vi "cRIO_MAC.vi"() -> (0 "MAC Address":string, 1 "Personality":string)   [LabVIEW 2016]
panel:
  out "File Text":string
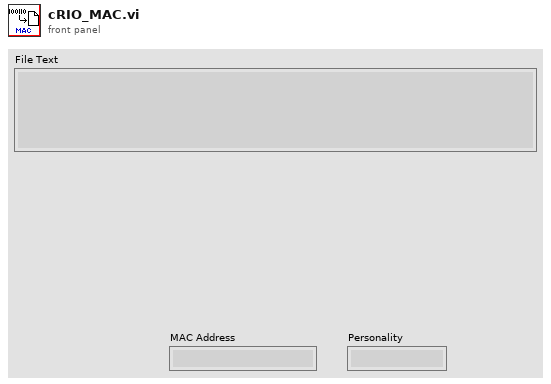
[diagram p1: front panel]
types:
  T1 = enum16{"open", "replace", "create", "open or create", "replace or create", "replace or create with confirmation"}
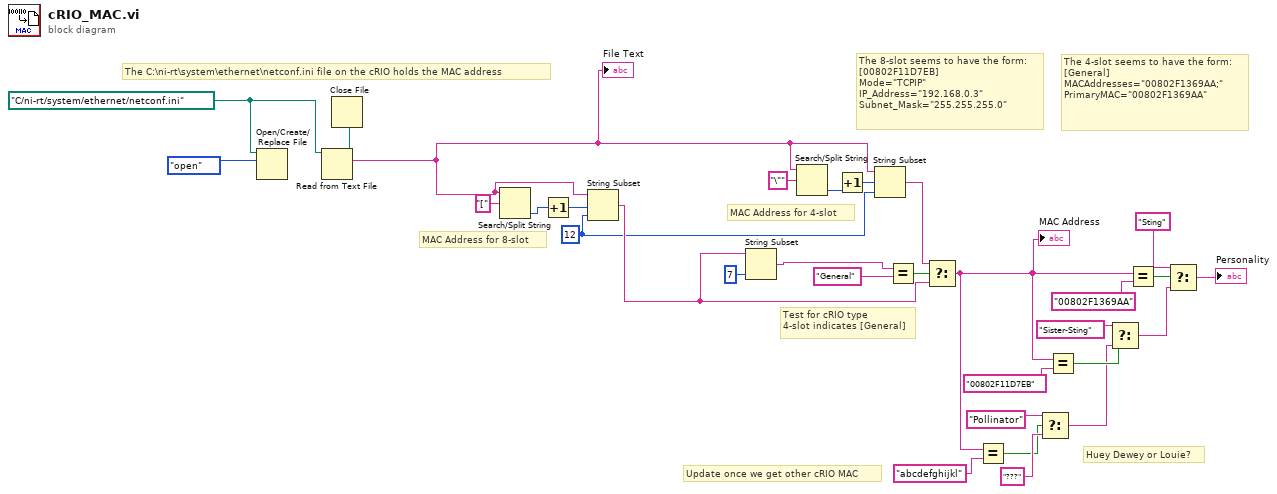
[diagram p0: block diagram]
diagram:
  w10 = path "C:/ni-rt/system/ethernet/netconf.ini" ("datalog path (use dialog)")
  w21 = 12 ("length (rest)")
  # "Update once we get other cRIO MAC"
  # "MAC Address for 8-slot"
  # "Huey Dewey or Louie?"
  # "MAC Address for 4-slot"
  # "The 4-slot seems to have the form:\n[General]\nMACAddresses=\"00802F1369AA;\"\nPrimaryMAC=\"00802F1369AA\""
  # "The 8-slot seems to have the form:\n[00802F11D7EB]\nMode=\"TCPIP\"\nIP_Address=\"192.168.0.3\"\nSubnet_Mask=\"255.255.255.0\""
  # "The C:\\ni-rt\\system\\ethernet\\netconf.ini file on the cRIO holds the MAC address"
  # "Test for cRIO type\n4-slot indicates [General]"
  n1 = Open/Create/Replace File(file path (use dialog)=w10, operation (0:open)=T1."open") -> ()  [unwired: 1 in, 6 out]
  n2 = Read from Text File(file (use dialog)=w10) -> (refnum out=w8:refnum<file>, text=w7:string)  [unwired: 3 in, 2 out]
  "File Text" <- w7
  n3 = Close File(refnum=w8) -> ()  [unwired: 1 in, 2 out]
  n4 = Search/Split String(string=w7, search string/char (-)="[") -> (offset of match=w30:i32)  [unwired: 1 in, 2 out]
  n5 = Increment(x=w30) -> (x+1=w31:i32)
  n6 = String Subset(string=w7, offset (0)=w31, length (rest)=w21) -> (substring=w25:string)
  n7 = String Subset(string=w25, length (rest)=7 ("length (rest)")) -> (substring=w28:string)  [unwired: 1 in]
  n8 = Search/Split String(string=w7, search string/char (-)="\"") -> (offset of match=w24:i32)  [unwired: 1 in, 2 out]
  n9 = Increment(x=w24) -> (x+1=w22:i32)
  n10 = String Subset(string=w7, offset (0)=w22, length (rest)=w21) -> (substring=w23:string)
  n11 = Equal?(x=w28, y="General") -> (x = y?=w26:bool)
  n12 = Select(t=w23, s=w26, f=w25) -> (s? t:f=w1:string)
  "MAC Address" <- w1
  n13 = Equal?(x=w1, y="abcdefghijkl") -> (x = y?=w4:bool)
  n14 = Select(t="Pollinator", s=w4, f="???") -> (s? t:f=w2:string)
  n15 = Equal?(x=w1, y="00802F11D7EB") -> (x = y?=w14:bool)
  n16 = Select(t="Sister-Sting", s=w14, f=w2) -> (s? t:f=w13:string)
  n17 = Equal?(x=w1, y="00802F1369AA") -> (x = y?=w17:bool)
  n18 = Select(t="Sting", s=w17, f=w13) -> (s? t:f=→"Personality":string)
